vi "IO_DataQ_GetCorrections.vi"(10 "index (row)":i32, 11 "Cal Array":dbl[][](array[numeric])) -> (3 "Array":dbl[](array[numeric]))   [LabVIEW 2024]
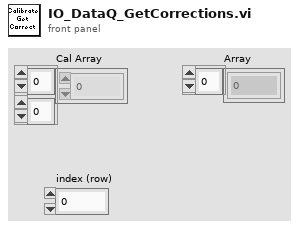
[diagram p1: front panel]
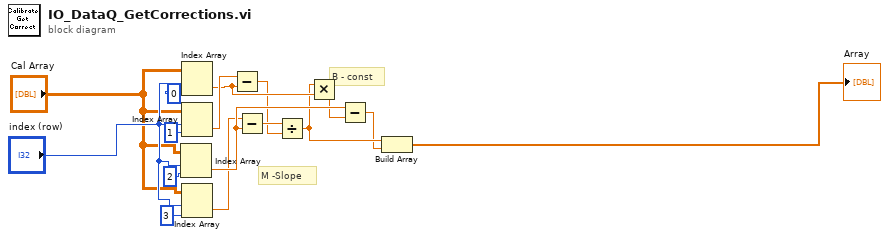
[diagram p0: block diagram]
diagram:
  # "B - const"
  # "M -Slope"
  n1 = Index Array(array="Cal Array", index (row)="index (row)", index (col)=2 ("disabled index (col)")) -> (element=w16:dbl)
  n2 = Index Array(array="Cal Array", index (row)="index (row)", index (col)=0 ("disabled index (col)")) -> (element=w13:dbl)
  n3 = Index Array(array="Cal Array", index (row)="index (row)", index (col)=1 ("disabled index (col)")) -> (element=w14:dbl)
  n4 = Index Array(array="Cal Array", index (row)="index (row)", index (col)=3 ("disabled index (col)")) -> (element=w15:dbl)
  n5 = Subtract(x=w14, y=w13) -> (x-y=w7:dbl)
  n6 = Subtract(x=w15, y=w16) -> (x-y=w8:dbl)
  n7 = Divide(x=w8, y=w7) -> (x/y=w12:dbl)
  n8 = Multiply(x=w12, y=w13) -> (x*y=w9:dbl)
  n9 = Subtract(x=w16, y=w9) -> (x-y=w10:dbl)
  n10 = Build Array(w12, w10) -> (→"Array":dbl[])
